vi "Assert Always.vi"(11 "Label":string) -> (0 "error out":errorcluster)   [LabVIEW 2013]
uses:
  classes/Assert/Assert.lvclass
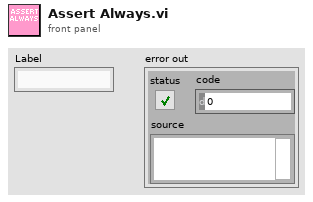
[diagram p1: front panel]
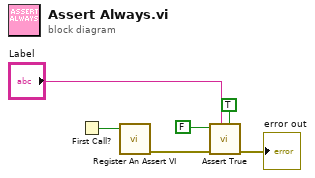
[diagram p0: block diagram]
diagram:
  n1 = First Call?() -> (First Call?: T/F=w5:bool)
  n2 = call "Register An Assert VI.vi"("first call?"=w5) -> ("error out"=w4:errorcluster)  [unwired: 10 in]
  n3 = call "Assert True.vi"("Assert Only? (F)"=TRUE, "Label"="Label", "error in (no error)"=w4, "True?"=FALSE) -> ("error out"=→"error out":errorcluster)  [unwired: 7 in]
